vi "AlliGator Select FLI Dataset Channel Name.vi"(8 "Error In":errorcluster, 9 "Channel Names":string[](array[string]), 11 "Input Message":string) -> (0 "Error Out":errorcluster, 1 "Cancelled?":bool, 2 "Channel Arithmetic":T1, 3 "Selected Channel":u16)   [LabVIEW 2021, in "AlliGator Dual-Channel Datasets.lvlib"]
doc: "Dialog window to select which SS3 channel to display."
uses:
  Settings/AlliGator Gate Arithmetic.ctl
  AlliGator Dual-Channel Datasets.lvlib
  Settings/AlliGator Settings.lvlib
panel:
  in  "Channel Arithmetic":T1
  in  "Channel Type":u16(ring) items=["Bottom INT Gate", "Bottom G2 Gate"]
  out "Message":string
  in  "Cancel":bool
  in  "OK":bool
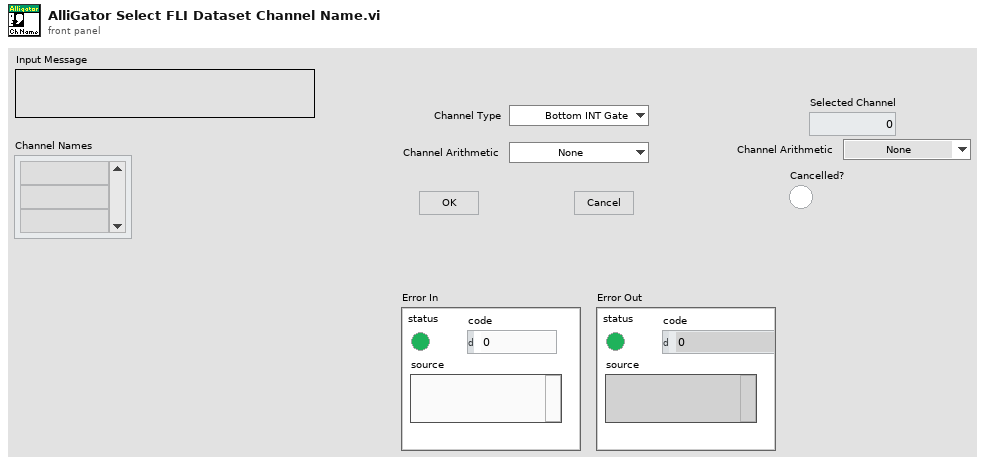
[diagram p1: front panel]
types:
  T1 = typedef "AlliGator Settings.lvlib/AlliGator Gate Arithmetic.ctl" = enum16{"None", "INT-G2", "G2/INT*<INT>", "(1 - G2/INT)*<INT>"}
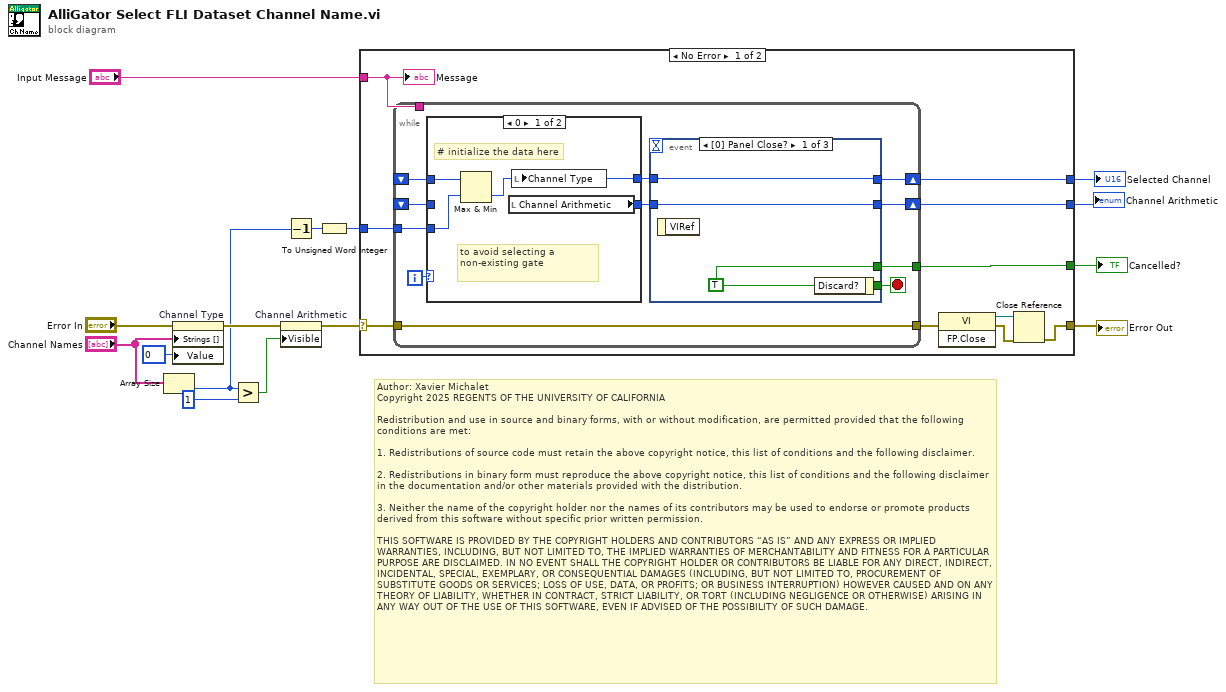
[diagram p0: block diagram]
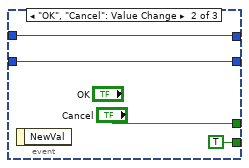
[diagram p3: hidden frame]
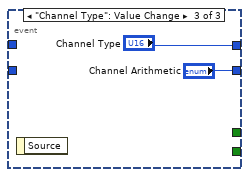
[diagram p4: hidden frame]
diagram:
  w4 = u16 0 items=[""] ("Gate Type")
  # "Author: Xavier Michalet\nCopyright 2025 REGENTS OF THE UNIVERSITY OF CALIFORNIA\n\nRedistribution and use in source and binary forms, with or without modification, are permitted provided that the following conditions are met:\n\n1. Redistributions of source code must retain the above copyright notice, this list of conditions and the following disclaimer.\n\n2. Redistributions in binary form must reproduce the above copyright notice, this list of conditions and the following disclaimer in the documentation and/or other materials provided with the distribution.\n\n3. Neither the name of the copyright holder nor the names of its contributors may be used to endorse or promote products derived from this software without specific prior written permission.\n\nTHIS SOFTWARE IS PROVIDED BY THE COPYRIGHT HOLDERS AND CONTRIBUTORS “AS IS” AND ANY EXPRESS OR IMPLIED WARRANTIES, INCLUDING, BUT NOT LIMITED TO, THE IMPLIED WARRANTIES OF MERCHANTABILITY AND FITNESS FOR A PARTICULAR PURPOSE ARE DISCLAIMED. IN NO EVENT SHALL THE COPYRIGHT HOLDER OR CONTRIBUTORS BE LIABLE FOR ANY DIRECT, INDIRECT, INCIDENTAL, SPECIAL, EXEMPLARY, OR CONSEQUENTIAL DAMAGES (INCLUDING, BUT NOT LIMITED TO, PROCUREMENT OF SUBSTITUTE GOODS OR SERVICES; LOSS OF USE, DATA, OR PROFITS; OR BUSINESS INTERRUPTION) HOWEVER CAUSED AND ON ANY THEORY OF LIABILITY, WHETHER IN CONTRACT, STRICT LIABILITY, OR TORT (INCLUDING NEGLIGENCE OR OTHERWISE) ARISING IN ANY WAY OUT OF THE USE OF THIS SOFTWARE, EVEN IF ADVISED OF THE POSSIBILITY OF SUCH DAMAGE."
  n1 = Array Size(array="Channel Names") -> (size(s)=w3:i32)
  n2 = property on="Channel Type" class="Ring (strict)"(error in="Error In", "Strings []"="Channel Names", "Value"=w4) -> (error out=w6:errorcluster)  [unwired: 1 in, 1 out]
  n3 = Greater?(x=w3, y=1) -> (0:w7:bool)
  n4 = property on="Channel Arithmetic" class="Enum (strict)"(error in=w6, "Visible"=w7) -> (error out=w5:errorcluster)  [unwired: 1 in, 1 out]
  n5 = Decrement(x=w3) -> (x-1=w2:i32)
  n6 = To Unsigned Word Integer(number=w2) -> (unsigned 16bit integer=w1:u16)
  n7 = case shown="No Error" w5 {
    selector: w5 -> [w19 w52]
    tunnel: [w25 _] -> w15
    tunnel: [w24 _] -> w14
    tunnel: "Input Message" -> [w23 _]
    tunnel: [w20 w52] -> w12
    tunnel: [w17 _] -> w10
    tunnel: w1 -> [w16 _]
    frame No Error {
      n8 = while {
        tunnel: [w35] -> w25
        shift-right: [w32] -> w24
        shift-left: _ -> [w33]
        tunnel: w23 -> [_]
        tunnel: w19 -> [w30]
        tunnel: [w30] -> w18
        shift-right: [w29] -> w17
        shift-left: _ -> [w27]
        tunnel: w16 -> [w26]
        i -> [w34]
        stop <- w36 stop-if-true
        n9 = case shown="0" w34 {
          tunnel: w33 -> [w40 w42]
          tunnel: [w37 w42] -> w31
          tunnel: [w39 w41] -> w28
          tunnel: w27 -> [_ w41]
          tunnel: w26 -> [w38 _]
          frame 0 {
            # "to avoid selecting a non-existing gate"
            # "# initialize the data here"
            n10 = Max & Min(x=w40, y=w38) -> (min(x,y)=w37:u16)  [unwired: 1 out]
            n11 = local read "Channel Arithmetic"() -> (w39:T1)
            n12 = local write "Channel Type"(w37) -> ()
          }
          frame 1, Default {
          }
        }
        n13 = event shown="[0] Panel Close?" {
          selector: _ -> [_ _ _]
          dyn-events: _ -> [_ _ _]
          timeout: _ -> [_ _ _]
          tunnel: [w45 TRUE ("Discard?") _] -> w36
          tunnel: [w45 "Cancel" _] -> w35
          tunnel: [w44 w47 "Channel Type"] -> w32
          tunnel: w31 -> [w44 w47 _]
          tunnel: [w43 w46 "Channel Arithmetic"] -> w29
          tunnel: w28 -> [w43 w46 _]
          event Panel Close? {
            w45 = TRUE ("Discard?")
            n14 = event-data() -> ()  [unwired: 1 in, 1 out]
            n15 = event-data("Discard?"=w45) -> ()  [unwired: 1 in, 1 out]
          }
          event "OK", "Cancel": Value Change {
            n16 = event-data() -> ()  [unwired: 1 in, 1 out]
          }
          event "Channel Type": Value Change {
            n17 = event-data() -> ()  [unwired: 1 in, 1 out]
          }
        }
      }
      n18 = invoke class="VI" method="FP.Close"(error in=w18) -> (reference out=w22:refnum<vi>, error out=w21:errorcluster)  [unwired: 2 in, 1 out]
      n19 = Close Reference(reference=w22, error in (no error)=w21) -> (error out=w20:errorcluster)
      "Message" <- w23
    }
    frame Error {
    }
  }
  "Selected Channel" <- w14
  "Cancelled?" <- w15
  "Error Out" <- w12
  "Channel Arithmetic" <- w10
